vi "Configure LAN.vi"(6 "Subnet Mask (255.255.255.0)":string="255.255.255.0", 7 "Gateway Address (0.0.0.0)":string="0.0.0.0", 8 "error in (no error)":errorcluster, 9 "IP Address (192.168.0.2)":string="192.168.0.2", 10 "LAN Configuration Method (0: Auto)":i32(ring) items=["Auto", "Manual"], 11 "VISA resource name":refnum<visa-resource-name>) -> (0 "error out":errorcluster, 3 "VISA resource name out":refnum<visa-resource-name>)   [LabVIEW 2015, in "Keithley 2600 Series.lvlib"]
doc: "Configures the basic settings of the LAN interface."
uses:
  Keithley 2600 Series.lvlib
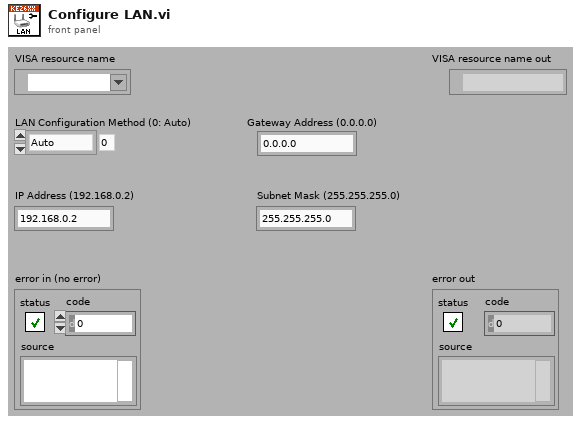
[diagram p1: front panel]
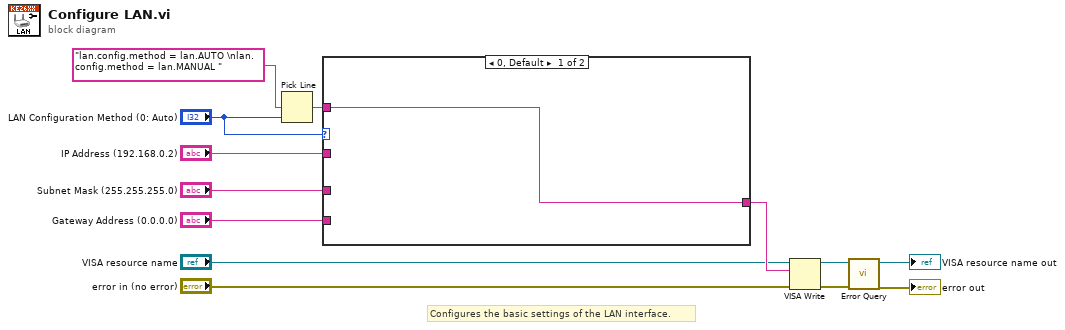
[diagram p0: block diagram]
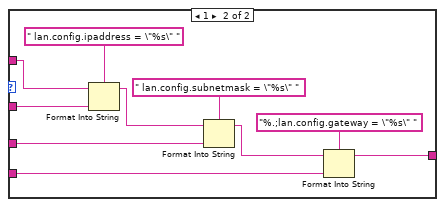
[diagram p2: hidden frame]
diagram:
  # "Configures the basic settings of the LAN interface."
  n1 = Pick Line(multi-line string="lan.config.method = lan.AUTO \nlan.config.method = lan.MANUAL ", line index="LAN Configuration Method (0: Auto)") -> (output string=w2:string)  [unwired: 1 in]
  n2 = case shown="0, Default" "LAN Configuration Method (0: Auto)" {
    tunnel: "IP Address (192.168.0.2)" -> [_ w23]
    tunnel: "Subnet Mask (255.255.255.0)" -> [_ w20]
    tunnel: "Gateway Address (0.0.0.0)" -> [_ w18]
    tunnel: [w14 w17] -> w9
    tunnel: w2 -> [w14 w16]
    frame 0, Default {
    }
    frame 1 {
      n3 = Format Into String(format string=" lan.config.ipaddress = \"%s\" ", initial string=w16, w23) -> (resulting string=w22:string)  [unwired: 1 in, 1 out]
      n4 = Format Into String(format string=" lan.config.subnetmask = \"%s\" ", initial string=w22, w20) -> (resulting string=w15:string)  [unwired: 1 in, 1 out]
      n5 = Format Into String(format string="%.;lan.config.gateway = \"%s\" ", initial string=w15, w18) -> (resulting string=w17:string)  [unwired: 1 in, 1 out]
    }
  }
  n6 = VISA Write(VISA resource name="VISA resource name", write buffer=w9, error in (no error)="error in (no error)") -> (VISA resource name out=w6:refnum<visa-resource-name>, error out=w5:errorcluster)  [unwired: 1 out]
  n7 = call "Error Query.vi"("error in (no error)"=w5, "VISA resource name"=w6) -> ("error out"=→"error out":errorcluster, "VISA resource name out"=→"VISA resource name out":refnum<visa-resource-name>)  [unwired: 6 in, 2 out]
